vi "Get VIs Paths by pattern.vi"(8 "error in":errorcluster, 10 "pattern":string, 11 "Library in":refnum<vi>) -> (0 "error out":errorcluster, 2 "All Files in Dir":path[](array[path]), 3 "Library out":refnum<vi>)   [LabVIEW 2019, in "Panther Dashboard.lvlib"]
uses:
  Panther Dashboard.lvlib
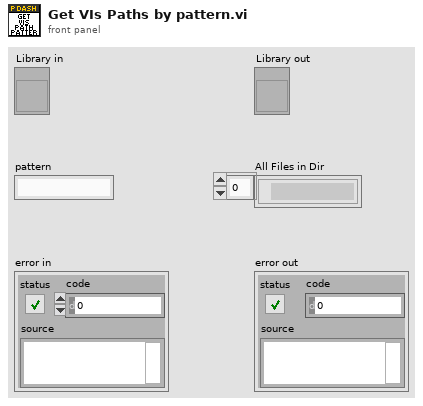
[diagram p1: front panel]
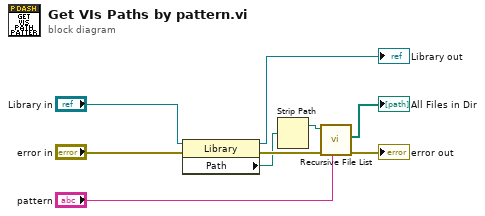
[diagram p0: block diagram]
diagram:
  n1 = property class="Library"(reference="Library in", error in="error in") -> (reference out=→"Library out":refnum<vi>, error out=w7:errorcluster, "Path"=w5:path)
  n2 = Strip Path(path=w5) -> (stripped path=w2:path)  [unwired: 1 out]
  n3 = call <vilib>:"Recursive File List.vi"("pattern"="pattern", "error in (no error)"=w7, "Folder Path"=w2) -> ("error out"=→"error out":errorcluster, "All Files in Dir"=→"All Files in Dir":path[])  [unwired: 4 in, 3 out]
